vi "Send Command Response.vi"(0 "LVx - Template Command in":refnum<class "LVx - Template Command.lvclass">, 11 "error in (no error)":errorcluster) -> (4 "LVx - Template Command out":refnum<class "LVx - Template Command.lvclass">, 15 "error out":errorcluster)   [LabVIEW 2011, in "LVx.lvlib" / "LVx - Template Command.lvclass"]
uses:
  LVx - Template Command.lvclass
  LVx.lvclass
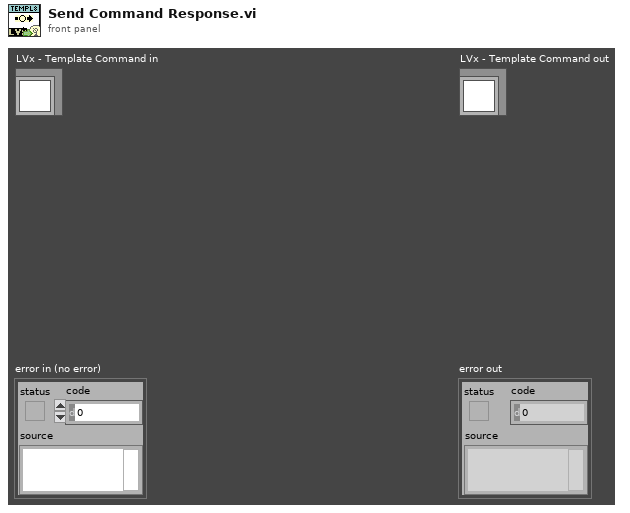
[diagram p1: front panel]
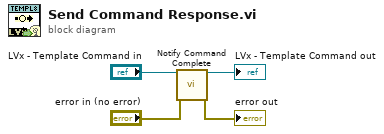
[diagram p0: block diagram]
diagram:
  n1 = call "Notify Command Complete.vi"("LVx.lvlib:LVx.lvclass"="LVx - Template Command in", "error in (no error)"="error in (no error)") -> ("LVx.lvclass out"=→"LVx - Template Command out":refnum<class "LVx - Template Command.lvclass">, "error out"=→"error out":errorcluster)  [unwired: 12 in]
